vi "BPN Test.vi"() -> ()   [LabVIEW 2015]
uses:
  Controls/Advanced Filter XCtl/Advanced Filter XCtl.xctl
  Waveform VIs/Noise VIs/Noise Params.ctl
  Controls/Level XCtl/Level Data.ctl
  Controls/Level XCtl/Level Units.ctl
  Controls/Level XCtl/Level XCtl.xctl
panel:
  out "Scale Factor":dbl
  in  "Cal File":path=path "C:/Data/XYZ DATA/XYZ999/RightPrimary.calib"
  out "Max Level":dbl
  in  "Level":T1={"Level"=0.0, "Units"=enum."dB SPL", "Max"=0.0, "Multiplier"=0.0, "Cal File"=path "", "Cal"={"Freq (Hz)"=[], "Mag (dB SPL)"=[], "Phase (deg)"=[]}}
  in  "Noise Params":T3
  in  "Sampling rate (Hz)":dbl=100000.0
  in  "Filter":T5(xcontrol)={"Type"=enum."Bandpass", "CF (kHz)"=4.0, "BW (kHz)"=0.333333, "Cascade"=FALSE, "Quadrature"=FALSE, "Scale Factor"=0.0, "Stages"=[], "Class"=enum."Elliptic", "Order"=0, "BWUnits"=enum."Octaves"}
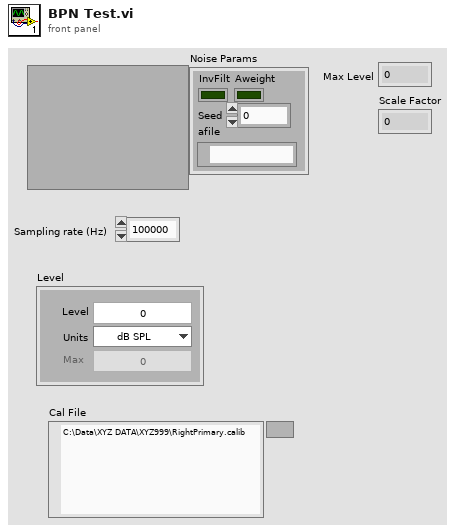
[diagram p1: front panel]
types:
  T1 = typedef "Level XCtl.xctl/Level Data.ctl" = cluster{"Level":dbl, "Units":T2, "Max":dbl, "Multiplier":dbl, "Cal File":path, "Cal":cluster{"Freq (Hz)":dbl[], "Mag (dB SPL)":dbl[], "Phase (deg)":dbl[]}}
  T2 = typedef "Level Units.ctl" = enum16{"dB atten", "dB SPL", "dB re 1 Vrms", "dB V/Hz½", "mW", "dB HL", "Volts", "dB mW"}
  T3 = typedef "Noise Params.ctl" = cluster{"InvFilt":bool, "Noise":dbl[], "CurPt":i32, "Aweight":bool, "Seed":i32, "afile":path}
  T4 = typedef "Filter-Bandwidth Units.ctl" = enum16{"Linear", "Octaves", "Min-Max"}
  T5 = cluster{"Type":enum16{"Lowpass", "Highpass", "Bandpass", "Bandstop", "OFF"}, "CF (kHz)":dbl, "BW (kHz)":dbl, "Cascade":bool, "Quadrature":bool, "Scale Factor":dbl, "Stages":cluster{"IIR Filter":cluster{"filter structure":enum32{"IIR 2nd Order", "IIR 4th Order"}, "Reverse Coefficients":dbl[], "Forward Coefficients":dbl[]}, "State":dbl[]}[], "Class":enum16{"Elliptic", "Butterworth"}, "Order":i32, "BWUnits":T4}
  T6 = typedef "Advanced Filter XCtl.xctl/Filter Data.ctl" = cluster{"Type":enum16{"Lowpass", "Highpass", "Bandpass", "Bandstop", "OFF"}, "CF (kHz)":dbl, "BW (kHz)":dbl, "Cascade":bool, "Quadrature":bool, "Scale Factor":dbl, "Stages":cluster{"IIR Filter":cluster{"filter structure":enum32{"IIR 2nd Order", "IIR 4th Order"}, "Reverse Coefficients":dbl[], "Forward Coefficients":dbl[]}, "State":dbl[]}[], "Class":enum16{"Elliptic", "Butterworth"}, "Order":i32, "BWUnits":T4}
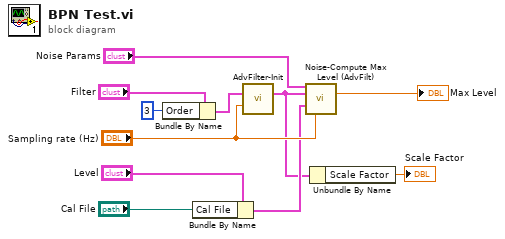
[diagram p0: block diagram]
diagram:
  n1 = Bundle By Name(cluster="Filter", "Order"=3) -> (w9:T5)
  n2 = Bundle By Name(cluster="Level", "Cal File"="Cal File") -> (w4:T1)
  n3 = call "AdvFilter-Init.vi"("Filter"=w9, "Sampling rate (Hz)"="Sampling rate (Hz)") -> ("Filter out"=w2:T6)  [unwired: 12 in, 1 out]
  n4 = call "Noise-Compute Max Level (AdvFilt).vi"("Noise Params"="Noise Params", "Filter XCtl"=w2, "Level"=w4, "Sampling Rate (Hz)"="Sampling rate (Hz)") -> ("Max Level"=→"Max Level":dbl)  [unwired: 9 in, 2 out]
  n5 = Unbundle By Name(w2) -> ("Scale Factor"=→"Scale Factor":dbl)
